vi "Write and Read Multiple Holding Registers1.vi"(4 "read count":u16, 6 "read operation starting address":u16, 7 "Unit_ID":T1, 8 "error in (no error)":errorcluster, 9 "values to write":u16[](array[numeric]), 10 "write operation starting address":u16, 11 "Modbus master in":refnum<class "TCP.lvclass">) -> (0 "error out":errorcluster, 1 "values read":u16[](array[numeric]), 3 "Modbus master out":refnum<class "TCP.lvclass">)   [LabVIEW 2019, in "NI_modbus_upd.lvlib"]
doc: "Writes and reads values to and from contiguous holding registers. This VI performs the write operation before the read operation. The maximum number of holding registers this VI can write is 121. The maximum number of holding registers this VI can read is 125."
uses:
  NI_modbus_upd.lvlib
  TCP/TCP.lvclass
  Ctl/Unit_ID.ctl
  TCP/TCP.lvclass/TCP.ctl
  Utility/Bytes to U16s1.vi
  Function code mismatch error1.vi
  Error Generator1.vi
  <vilib>/Modbus/subvis/Utility/U16s to Bytes.vi
  Modbus Data Unit (PDU)/Construct PDU1.vi
  Read ADU Packet Master.vi
  Write ADU Packet Master.vi
  Modbus Data Unit (PDU)/Unflatten to PDU1.vi
  TCP/Protocol Read.vi
  TCP/Protocol Write.vi
  <vilib>/Utility/error.llb/Error Cluster From Error Code.vi
  Modbus Data Unit (PDU)/Deconstruct PDU1.vi
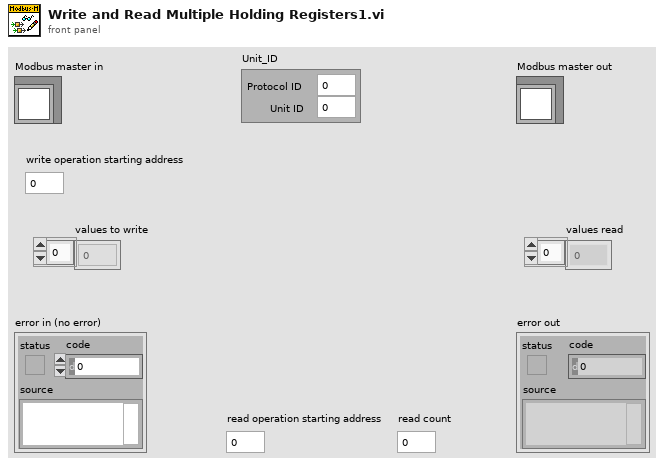
[diagram p1: front panel]
types:
  T1 = typedef "NI_modbus_upd.lvlib/Unit_ID.ctl" = cluster{"Protocol ID":u16, "Unit ID":u8}
  T2 = typedef "NI_modbus_upd.lvlib/MB Modbus Data Unit.ctl" = cluster{"function":T3, "Data":u8[]}
  T3 = typedef "NI_modbus_upd.lvlib/Function.ctl" = u8
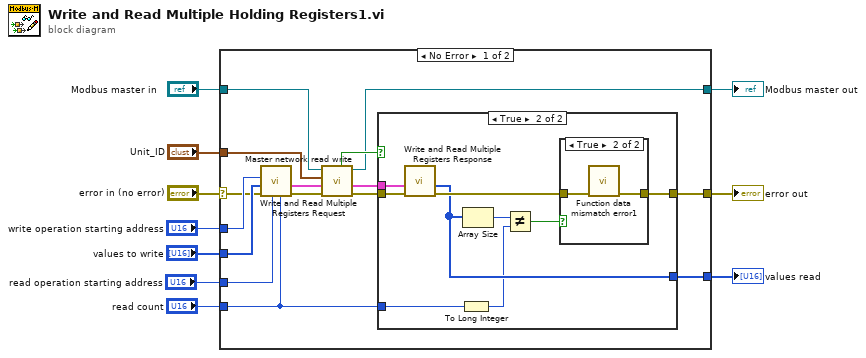
[diagram p0: block diagram]
diagram:
  n1 = case shown="No Error" "error in (no error)" {
    selector: "error in (no error)" -> [w11 w39]
    tunnel: "Modbus master in" -> [w14 w40]
    tunnel: [w16 w40] -> w9
    tunnel: [w24 w39] -> w8
    tunnel: "read count" -> [w22 _]
    tunnel: [w21 _] -> w5
    tunnel: "read operation starting address" -> [w20 _]
    tunnel: "values to write" -> [w19 _]
    tunnel: "write operation starting address" -> [w18 _]
    tunnel: "Unit_ID" -> [w13 _]
    frame No Error {
      n2 = call "Write and Read Multiple Registers Request.vi"("quantity to read"=w22, "read starting address"=w20, "error in (no error)"=w11, "write"=w19, "write starting address"=w18) -> ("error out"=w25:errorcluster, "Modbus data unit out"=w12:T2)  [unwired: 5 in]
      n3 = call "Master network read write.vi"("error in (no error)"=w25, "Modbus Data Unit"=w12, "Unit_ID"=w13, "TCP in"=w14) -> ("error out"=w23:errorcluster, "Modbus data unit out"=w15:T2, "TCP out"=w16:refnum<class "TCP.lvclass">, "PDU valid?"=w17:bool)  [unwired: 4 in]
      n4 = case shown="True" w17 {
        tunnel: [w26 w35] -> w24
        tunnel: w23 -> [w26 w34]
        tunnel: w22 -> [_ w30]
        tunnel: [_ w29] -> w21
        tunnel: w15 -> [_ w27]
        frame False {
        }
        frame True {
          n5 = call "Write and Read Multiple Registers Response.vi"("error in (no error)"=w34, "Modbus Data Unit in"=w27) -> ("error out"=w33:errorcluster, "registers"=w29:u16[])  [unwired: 7 in, 1 out]
          n6 = To Long Integer(number=w30) -> (32bit integer=w28:i32)
          n7 = Array Size(array=w29) -> (size(s)=w31:i32)
          n8 = Not Equal?(x=w31, y=w28) -> (x != y?=w32:bool)
          n9 = case shown="True" w32 {
            tunnel: [w36 w38] -> w35
            tunnel: w33 -> [w36 w37]
            frame False {
            }
            frame True {
              n10 = call "Function data mismatch error1.vi"("error in (no error)"=w37) -> ("error out"=w38:errorcluster)  [unwired: 10 in]
            }
          }
        }
      }
    }
    frame Error {
    }
  }
  "error out" <- w8
  "Modbus master out" <- w9
  "values read" <- w5
